vi "rhominus.vi"(10 "Array":dbl[](array[numeric]), 11 "Array 2":dbl[](array[numeric])) -> (3 "Array 3":dbl[](array[numeric]))   [LabVIEW 2019]
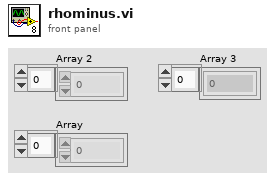
[diagram p1: front panel]
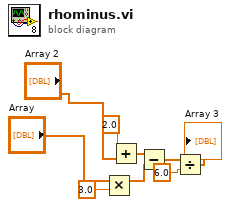
[diagram p0: block diagram]
diagram:
  n1 = Multiply(x="Array", y=3.0) -> (x*y=w2:dbl[])
  n2 = Add(x=2.0, y="Array 2") -> (x+y=w4:dbl[])
  n3 = Subtract(x=w4, y=w2) -> (x-y=w5:dbl[])
  n4 = Divide(x=w5, y=6.0) -> (x/y=→"Array 3":dbl[])
